vi "Stop Core.vi"(10 "final error code":i32, 11 "Core in":refnum<class "Core.lvclass">) -> (3 "Core out":refnum<class "Core.lvclass">)   [LabVIEW 2019, in "Core.lvlib" / "Core.lvclass"]
doc: "(<B>Filename</B>: Actor Framework.lvlib:Actor.lvclass:Stop Core.vi)\n\nDefines what the actor does before it stops. Use the <B>final error code</B> input to determine whether the actor shut down in response to an error.\n\nBy default, this method passes the Stop message along to all auto-stop nested actors. A descendant class may override this method to define additional behavior, such as shutting down any processes the actor initiated in its override of the Actor Core method."
uses:
  Core.lvclass
  ModuleAbstract/ModuleAbstract.lvclass
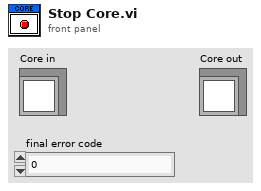
[diagram p1: front panel]
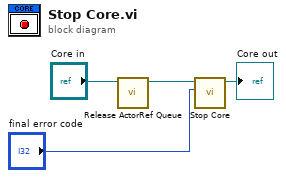
[diagram p0: block diagram]
diagram:
  n1 = call "Release ActorRef Queue.vi"("Core In"="Core in") -> ("Core Out"=w1:refnum<class "Core.lvclass">)  [unwired: 9 in, 1 out]
  n2 = call-parent "Stop Core.vi"("final error code"="final error code", "ModuleAbstract in"=w1) -> ("ModuleAbstract out"=→"Core out":refnum<class "Core.lvclass">)  [unwired: 9 in]
